vi "Create Store Array.vi"(4 "Columns to save":bool[](array[boolean])=[TRUE, TRUE, FALSE, FALSE, FALSE, FALSE, FALSE, FALSE, FALSE, FALSE, FALSE, FALSE]) -> (1 "Array":dbl[][](array[numeric]))   [LabVIEW 2013]
uses:
  Store Data Actions.ctl
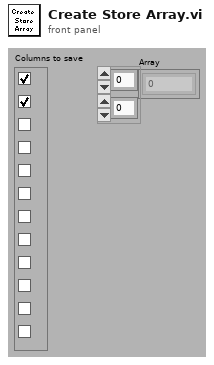
[diagram p1: front panel]
types:
  T1 = typedef "Store Data Actions.ctl" = enum16{"Init", "Set", "Add", "Add Array", "Read", "Row+N"}
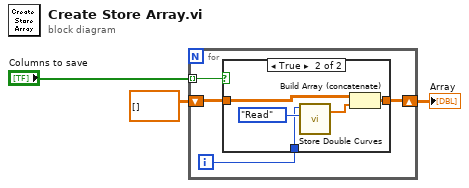
[diagram p0: block diagram]
diagram:
  n1 = for {
    shift-right: [w6] -> w1
    shift-left: dbl[][] [] -> [w5]
    tunnel: "Columns to save" -> [w4] mode=indexing
    i -> [w7]
    n2 = case shown="True" w4 {
      tunnel: w7 -> [_ w12]
      tunnel: [w8 w10] -> w6
      tunnel: w5 -> [w8 w9]
      frame False {
      }
      frame True {
        n3 = call "Store Double Curves.vi"("Action"=Store_Data_Actions."Read", "Curve Index"=w12) -> ("Array out"=w11:dbl[])  [unwired: 4 in, 1 out]
        n4 = Build Array (concatenate)(w9, w11) -> (w10:dbl[][])
      }
    }
  }
  "Array" <- w1
